vi "Read VI.vi"(8 "error in (no error)":errorcluster, 10 "VI Path (.vi)":path, 11 "VI Refnum":refnum<vi>) -> (0 "error out":errorcluster, 3 "Snippet":T1)   [LabVIEW 2022 SP3, in "VI-Snippet.lvlib"]
doc: "Saves a copy of <b>VI Refnum</b> to <b>VI Path (.vi)</b> and returns the snippet content."
uses:
  VI-Snippet.lvlib
  Snippet.ctl
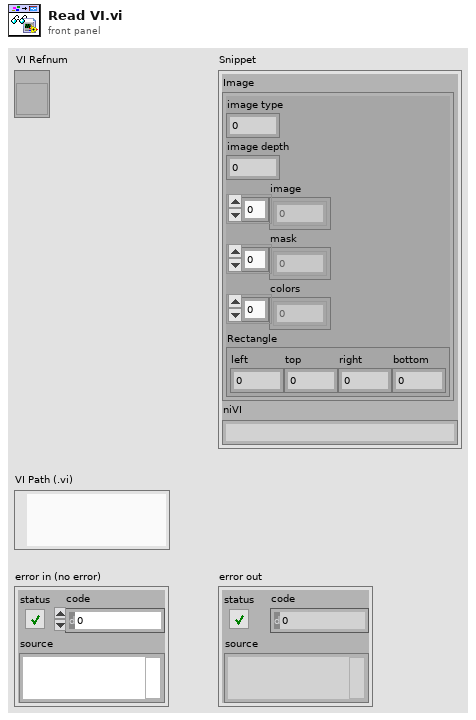
[diagram p1: front panel]
types:
  T1 = typedef "VI-Snippet.lvlib/Snippet.ctl" = cluster{"Image":cluster{"image type":i32, "image depth":i32, "image":u8[], "mask":u8[], "colors":u32[], "Rectangle":cluster{"left":i16, "top":i16, "right":i16, "bottom":i16}}, "niVI":string}
  T2 = cluster{"image type":i32, "image depth":i32, "image":u8[], "mask":u8[], "colors":u32[], "Rectangle":cluster{"left":i16, "top":i16, "right":i16, "bottom":i16}}
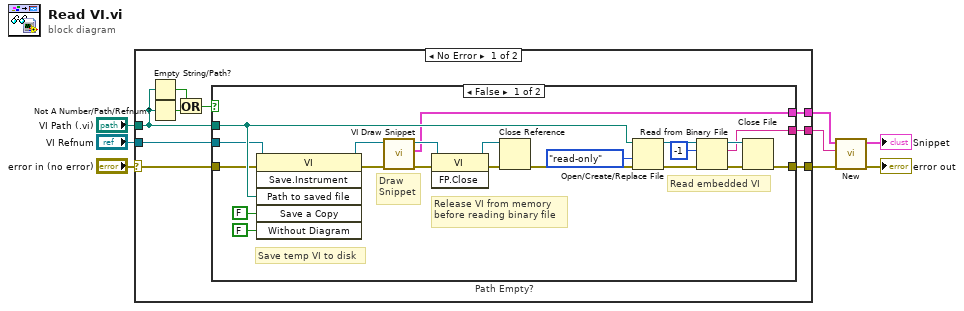
[diagram p0: block diagram]
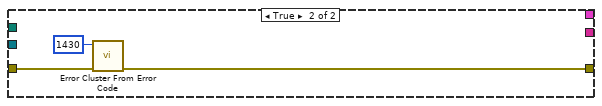
[diagram p2: hidden frame]
diagram:
  n1 = case shown="No Error" "error in (no error)" {
    selector: "error in (no error)" -> [w14 w42]
    tunnel: "VI Path (.vi)" -> [w10 _]
    tunnel: [w17 w42] -> w5
    tunnel: "VI Refnum" -> [w13 _]
    tunnel: [w16 _] -> w2
    tunnel: [w15 _] -> w3
    frame No Error {
      n2 = Empty String/Path?(string/path=w10) -> (empty?=w11:bool)
      n3 = Not A Number/Path/Refnum?(number/path/refnum=w10) -> (NaN/Path/Refnum?=w12:bool)
      n4 = Or(x=w11, y=w12) -> (x .or. y?=w9:bool)
      n5 = case "Path Empty?" shown="False" w9 {
        tunnel: w10 -> [w23 _]
        tunnel: [w22 w40] -> w17
        tunnel: [w21 _] -> w16
        tunnel: [w20 _] -> w15
        tunnel: w14 -> [w19 w41]
        tunnel: w13 -> [w18 _]
        frame False {
          # "Read embedded VI"
          # "Draw\nSnippet"
          # "Release VI from memory\nbefore reading binary file"
          # "Save temp VI to disk"
          n6 = invoke class="VI" method="Save.Instrument"(reference=w18, error in=w19, "Path to saved file"=w23, "Save a Copy"=FALSE, "Without Diagram"=FALSE) -> (reference out=w33:refnum<vi>, error out=w34:errorcluster)  [unwired: 1 in, 4 out]
          n7 = call "VI Draw Snippet.vi"("error in (no error)"=w34, "VI Refnum"=w33) -> ("error out"=w32:errorcluster, "Image Data"=w21:T2, "dup VI Refnum"=w31:refnum<vi>)  [unwired: 7 in]
          n8 = invoke class="VI" method="FP.Close"(reference=w31, error in=w32) -> (reference out=w35:refnum<vi>, error out=w36:errorcluster)  [unwired: 1 in, 1 out]
          n9 = Close Reference(reference=w35, error in (no error)=w36) -> (error out=w25:errorcluster)
          n10 = Open/Create/Replace File(file path (use dialog)=w23, error in=w25, access (0:read/write)=enum16{"read/write", "read-only", "write-only"}."read-only") -> (refnum out=w27:refnum<file>, error out=w26:errorcluster)  [unwired: 3 in, 1 out]
          n11 = Read from Binary File(8:w26, 10:-1 ("count (1)"), 11:w27) -> (0:w29:errorcluster, 2:w20:string, 3:w28:refnum<file>)  [unwired: 3 in, 1 out]
          n12 = Close File(refnum=w28, error in=w29) -> (error out=w22:errorcluster)  [unwired: 1 out]
        }
        frame True {
          n13 = call <vilib>:"Error Cluster From Error Code.vi"("error in (no error)"=w41, "error code (0)"=1430) -> ("error out"=w40:errorcluster)  [unwired: 7 in]
        }
      }
    }
    frame Error {
    }
  }
  n14 = call "New.vi"("error in (no error)"=w5, "niVI"=w3, "Image"=w2) -> ("error out"=→"error out":errorcluster, "VI Snippet out"=→"Snippet":T1)  [unwired: 7 in]
